vi "Make Filenames.vi"(7 "Category":string, 8 "error in (no error)":errorcluster, 9 "Suffix":string, 10 "# Columns":i16, 11 "iteration variable":i16) -> (0 "error out":errorcluster, 3 "Spectra filename":string)   [LabVIEW 2018]
doc: "Use this template to build a VI to use as a subVI."
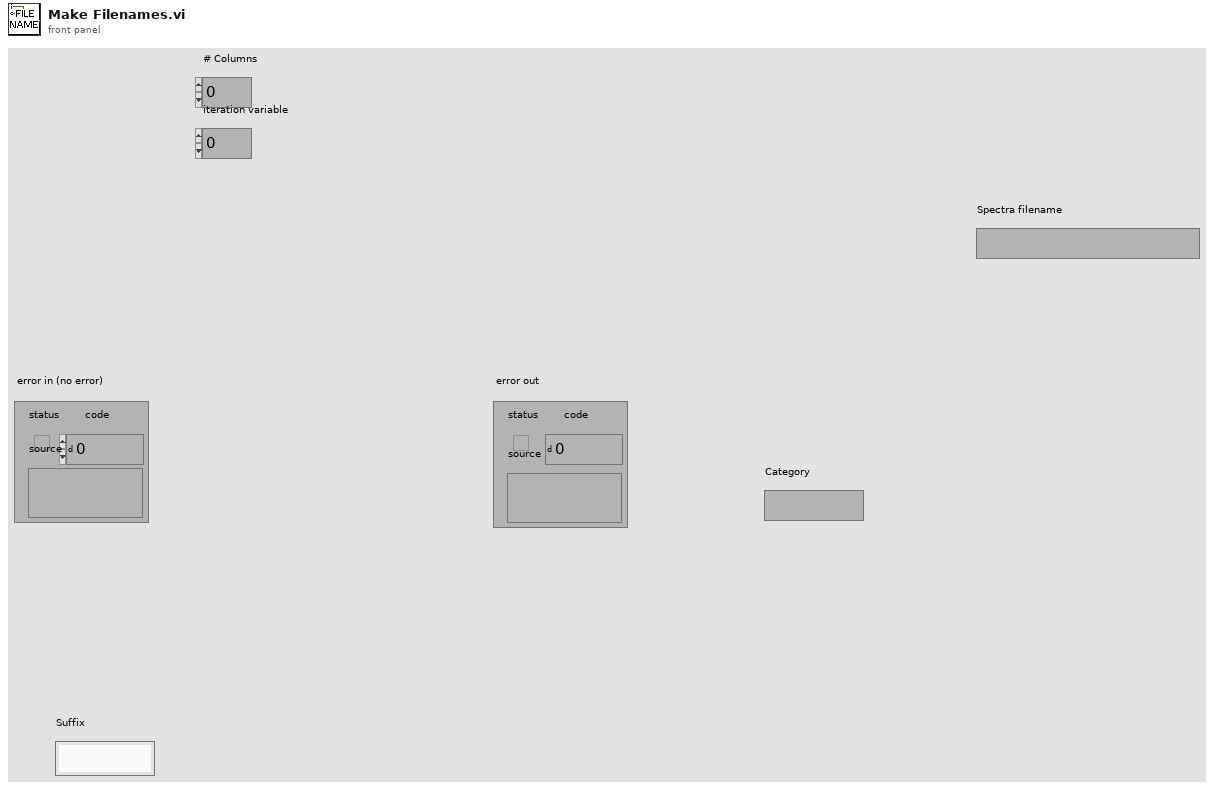
[diagram p1: front panel]
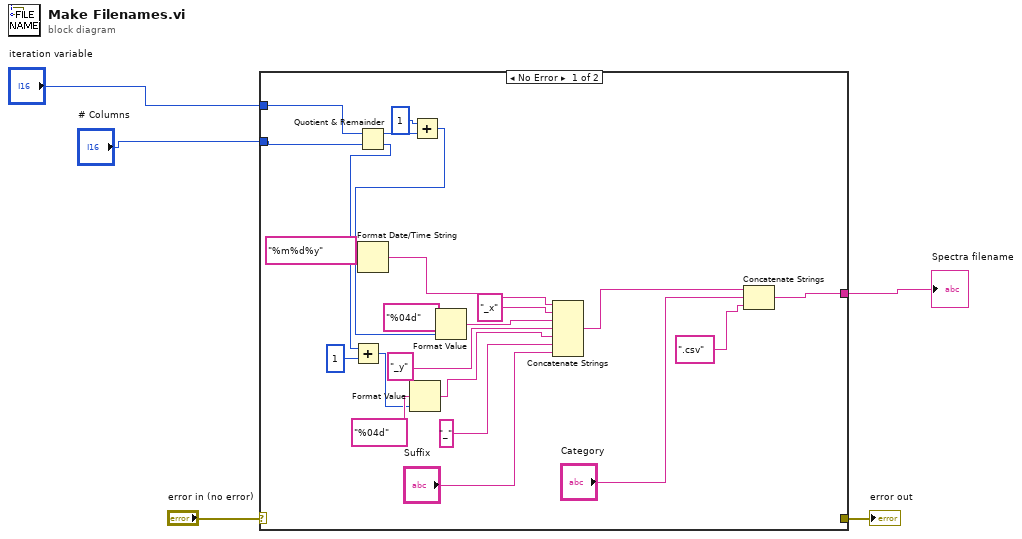
[diagram p0: block diagram]
diagram:
  n1 = case shown="No Error" "error in (no error)" {
    selector: "error in (no error)" -> [_ w28]
    tunnel: [_ w28] -> w4
    tunnel: "# Columns" -> [w16 _]
    tunnel: "iteration variable" -> [w15 _]
    tunnel: [w8 _] -> w1
    frame No Error {
      n2 = Quotient & Remainder(x=w15, y=w16) -> (x-y*floor(x/y)=w18:i16, floor(x/y)=w11:i16)
      n3 = Add(x=w11, y=i16 1) -> (x+y=w9:i16)
      n4 = Format Date/Time String(time format string (%c)="%m%d%y") -> (date/time string=w12:string)  [unwired: 2 in]
      n5 = Format Value(format string="%04d", value (0)=w9) -> (output string=w24:string)  [unwired: 1 in]
      n6 = Add(x=i16 1, y=w18) -> (x+y=w14:i16)
      n7 = Format Value(format string="%04d", value (0)=w14) -> (output string=w21:string)  [unwired: 1 in]
      n8 = Concatenate Strings(w12, "_x" ("string"), w21, "_y" ("string"), w24, "_" ("string"), "Suffix") -> (w27:string)
      n9 = Concatenate Strings(w27, "Category", ".csv" ("string")) -> (w8:string)
    }
    frame Error {
    }
  }
  "error out" <- w4
  "Spectra filename" <- w1
